vi "linear_ramp.vi"(10 "filter const (dx/dt)":dbl, 11 "input":dbl) -> (3 "output":dbl)   [LabVIEW 2012]
panel:
  # "dx is in input units\ndt is in seconds"
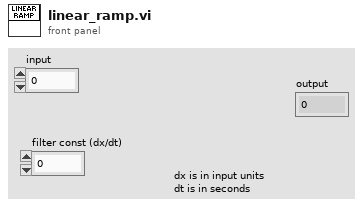
[diagram p1: front panel]
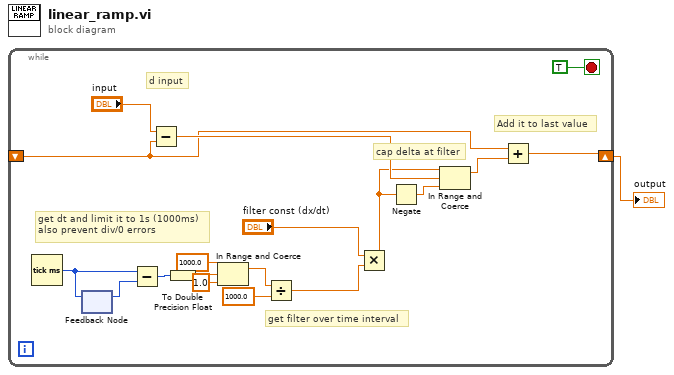
[diagram p0: block diagram]
diagram:
  n1 = while {
    shift-right: [w3] -> w1
    shift-left: _ -> [w2]
    stop <- TRUE stop-if-true
    # "Add it to last value"
    # "cap delta at filter"
    # "d input"
    # "get filter over time interval"
    # "get dt and limit it to 1s (1000ms)\nalso prevent div/0 errors"
    n2 = Tick Count (ms)() -> (millisecond timer value=w16:u32)
    n3 = feedback-in #1(w16) -> ()
    n4 = feedback #1() -> (w15:u32)  [unwired: 1 in]
    n5 = Subtract(x=w16, y=w15) -> (x-y=w14:u32)
    n6 = Subtract(x="input", y=w2) -> (x-y=w17:dbl)
    n7 = To Double Precision Float(number=w14) -> (double precision float=w13:dbl)
    n8 = In Range and Coerce(upper limit=1000.0, x=w13, lower limit=1.0) -> (coerced(x)=w9:dbl)  [unwired: 1 out]
    n9 = Divide(x=w9, y=1000.0) -> (x/y=w7:dbl)
    n10 = Multiply(x="filter const (dx/dt)", y=w7) -> (x*y=w5:dbl)
    n11 = Negate(x=w5) -> (-x=w6:dbl)
    n12 = In Range and Coerce(upper limit=w5, x=w17, lower limit=w6) -> (coerced(x)=w4:dbl)  [unwired: 1 out]
    n13 = Add(x=w2, y=w4) -> (x+y=w3:dbl)
  }
  "output" <- w1
